vi "clear connection.vi"(8 "error in (no error)":errorcluster, 11 "tcp server in":refnum<class "tcp connection.lvclass">) -> (0 "error out":errorcluster, 3 "tcp server out":refnum<class "tcp connection.lvclass">)   [LabVIEW 2014, in "tcp connection.lvclass"]
doc: "This vi will execute normally even if there is an incoming error."
uses:
  tcp connection.lvclass
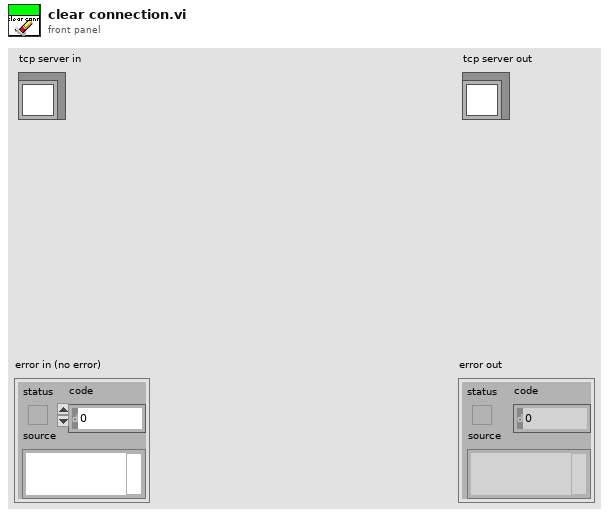
[diagram p1: front panel]
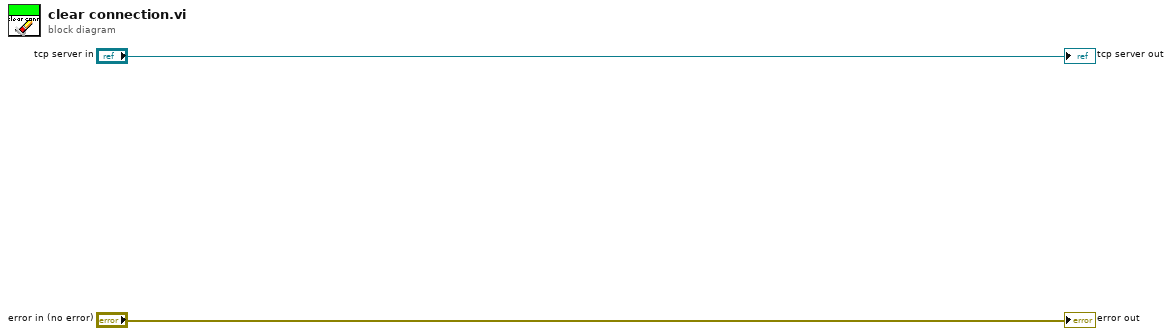
[diagram p0: block diagram]
diagram:
  "error out" <- "error in (no error)"
  "tcp server out" <- "tcp server in"
